vi "Odometry.vi"(0 "Enc0":dbl, 1 "Enc1":dbl, 2 "Enc2":dbl, 3 "Enc3":dbl, 4 "Az0":dbl, 5 "Az1":dbl, 6 "Az2":dbl, 7 "Az3":dbl, 8 "Heading":dbl, 9 "in SWERVE_DRIVE_ODOMETRY":T1={"POSE"={"TRANSLATION"={"X"=0.0, "Y"=0.0}, "ROTATION"={"VALUE"=0.0, "COS"=1.0, "SIN"=0.0}}, "GyroOffset"={"VALUE"=0.0, "COS"=1.0, "SIN"=0.0}, "PreviousAngle"={"VALUE"=0.0, "COS"=1.0, "SIN"=0.0}, "PrevModulePositions"=[], "NumModules"=0} {"PrevModulePositions"."Angle"."SIN" format="%13.4f"; "PrevModulePositions"."Angle"."COS" format="%13.4f"; "PrevModulePositions"."Angle"."VALUE" format="%13.4f"; "PreviousAngle"."SIN" format="%13.4f"; "PreviousAngle"."COS" format="%13.4f"; "PreviousAngle"."VALUE" format="%13.4f"; "GyroOffset"."SIN" format="%13.4f"; "GyroOffset"."COS" format="%13.4f"; "GyroOffset"."VALUE" format="%13.4f"; "POSE"."ROTATION"."SIN" format="%13.4f"; "POSE"."ROTATION"."COS" format="%13.4f"; "POSE"."ROTATION"."VALUE" format="%13.4f"; "POSE"."TRANSLATION"."Y" format="%14.3f"; "POSE"."TRANSLATION"."X" format="%14.3f"}) -> (20 "robot POSE":T2={"TRANSLATION"={"X"=0.0, "Y"=0.0}, "ROTATION"={"VALUE"=0.0, "COS"=1.0, "SIN"=0.0}} {"ROTATION"."SIN" format="%13.4f"; "ROTATION"."COS" format="%13.4f"; "ROTATION"."VALUE" format="%13.4f"; "TRANSLATION"."Y" format="%14.3f"; "TRANSLATION"."X" format="%14.3f"}, 21 "out SWERVE_DRIVE_ODOMETRY":T1={"POSE"={"TRANSLATION"={"X"=0.0, "Y"=0.0}, "ROTATION"={"VALUE"=0.0, "COS"=1.0, "SIN"=0.0}}, "GyroOffset"={"VALUE"=0.0, "COS"=1.0, "SIN"=0.0}, "PreviousAngle"={"VALUE"=0.0, "COS"=1.0, "SIN"=0.0}, "PrevModulePositions"=[], "NumModules"=0} {"PrevModulePositions"."Angle"."SIN" format="%13.4f"; "PrevModulePositions"."Angle"."COS" format="%13.4f"; "PrevModulePositions"."Angle"."VALUE" format="%13.4f"; "PreviousAngle"."SIN" format="%13.4f"; "PreviousAngle"."COS" format="%13.4f"; "PreviousAngle"."VALUE" format="%13.4f"; "GyroOffset"."SIN" format="%13.4f"; "GyroOffset"."COS" format="%13.4f"; "GyroOffset"."VALUE" format="%13.4f"; "POSE"."ROTATION"."SIN" format="%13.4f"; "POSE"."ROTATION"."COS" format="%13.4f"; "POSE"."ROTATION"."VALUE" format="%13.4f"; "POSE"."TRANSLATION"."Y" format="%14.3f"; "POSE"."TRANSLATION"."X" format="%14.3f"})   [LabVIEW 2020]
uses:
  <vilib>/Rock Robotics/WPI/ThirdParty/JAS_Junk/TrajLib/Trajectory_Library.lvlib
  <vilib>/Rock Robotics/WPI/ThirdParty/JAS_Junk/TrajLib/TypeDef/TRANSLATION2D.ctl
  <vilib>/Rock Robotics/WPI/ThirdParty/JAS_Junk/TrajLib/TypeDef/ROTATION2D.ctl
  <vilib>/Rock Robotics/WPI/ThirdParty/JAS_Junk/TrajLib/TypeDef/POSE2D.ctl
  <vilib>/Rock Robotics/WPI/ThirdParty/JAS_Junk/TrajLib/TypeDef/SWERVE_DRIVE_MODULE_POSITION.ctl
  <vilib>/Rock Robotics/WPI/ThirdParty/JAS_Junk/TrajLib/TypeDef/SWERVE_DRIVE_ODOMETRY.ctl
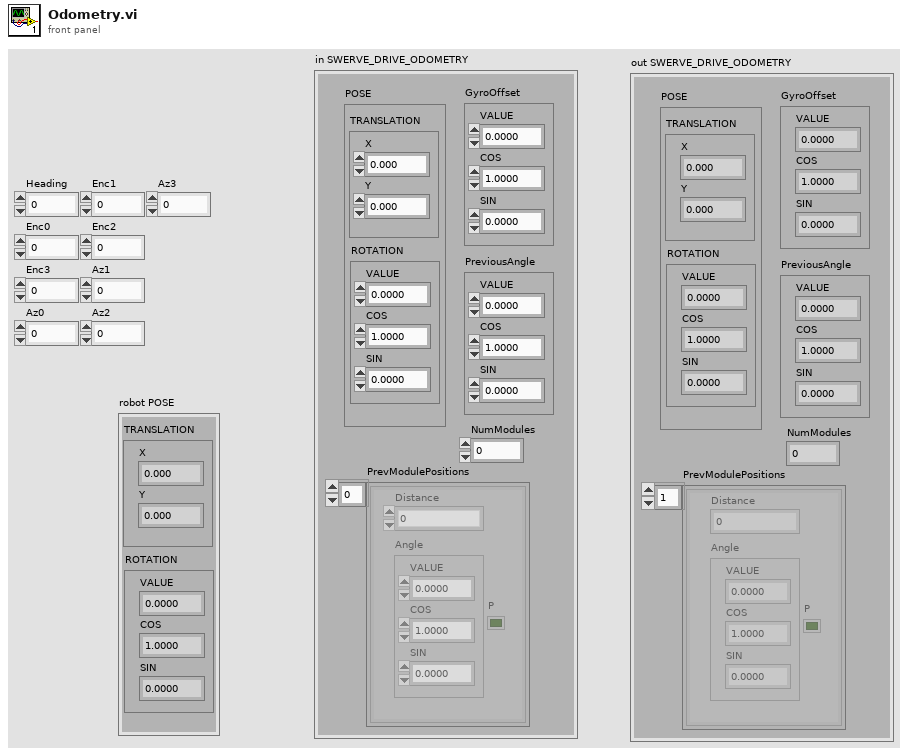
[diagram p1: front panel]
types:
  T1 = typedef "Trajectory_Library.lvlib/SWERVE_DRIVE_ODOMETRY.ctl" = cluster{"POSE":T2, "GyroOffset":T4, "PreviousAngle":T4, "PrevModulePositions":T5[], "NumModules":i32}
  T2 = typedef "Trajectory_Library.lvlib/POSE2D.ctl" = cluster{"TRANSLATION":T3, "ROTATION":T4}
  T3 = typedef "Trajectory_Library.lvlib/TRANSLATION2D.ctl" = cluster{"X":dbl, "Y":dbl}
  T4 = typedef "Trajectory_Library.lvlib/ROTATION2D.ctl" = cluster{"VALUE":dbl, "COS":dbl, "SIN":dbl}
  T5 = typedef "Trajectory_Library.lvlib/SWERVE_DRIVE_MODULE_POSITION.ctl" = cluster{"Distance":dbl, "Angle":T4, "P":bool}
  T6 = typedef "Trajectory_Library.lvlib/SWERVE_DRIVE_KINEMATICS.ctl" = cluster{"NumModules":i32, "InverseKinematics":T7, "ForwardKinematics":T7, "Modules":T3[], "PrevCoR":T3, "SavedModuleStates":T8[]}
  T7 = typedef "NI_Matrix.lvlib/RealMatrix.ctl" = dbl[][]
  T8 = typedef "Trajectory_Library.lvlib/SWERVE_DRIVE_MODULE_STATE.ctl" = cluster{"Speed":dbl, "Angle":T4}
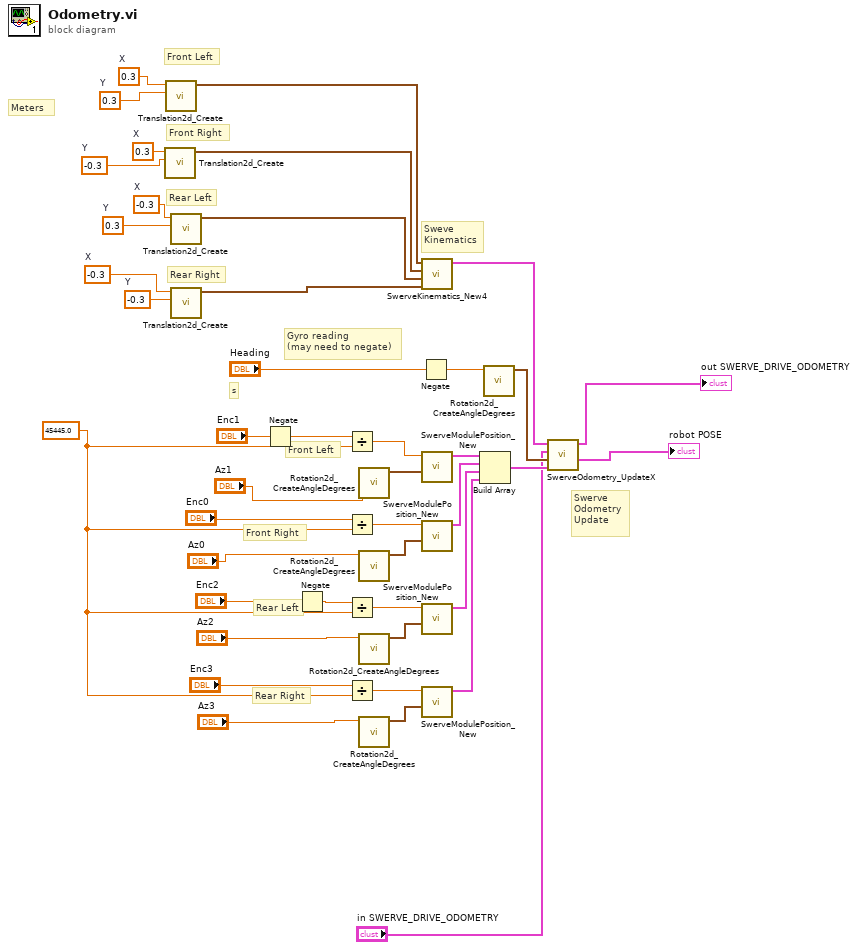
[diagram p0: block diagram]
diagram:
  w23 = 45445.0 ("y")
  w34 = -0.3  # X
  w35 = -0.3  # Y
  w32 = -0.3  # X
  w33 = 0.3  # Y
  w30 = 0.3  # X
  w31 = -0.3  # Y
  w28 = 0.3  # X
  w29 = 0.3  # Y
  # "s"
  # "Meters"
  # "Sweve\nKinematics"
  # "Rear Right"
  # "Rear Left"
  # "Front Right"
  # "Front Left"
  # "Swerve\nOdometry\nUpdate"
  # "Rear Right"
  # "Rear Left"
  # "Front Right"
  # "Front Left"
  # "Gyro reading\n(may need to negate)"
  n1 = call <vilib>:"Translation2d_Create.vi"("Y"=w31, "X"=w30) -> ("TRANSLATION"=w18:T3)  [unwired: 9 in]
  n2 = call <vilib>:"Translation2d_Create.vi"("Y"=w29, "X"=w28) -> ("TRANSLATION"=w19:T3)  [unwired: 9 in]
  n3 = call <vilib>:"Translation2d_Create.vi"("Y"=w33, "X"=w32) -> ("TRANSLATION"=w17:T3)  [unwired: 9 in]
  n4 = call <vilib>:"Translation2d_Create.vi"("Y"=w35, "X"=w34) -> ("TRANSLATION"=w16:T3)  [unwired: 9 in]
  n5 = Negate(x="Enc1") -> (-x=w2:dbl)
  n6 = Negate(x="Enc2") -> (-x=w1:dbl)
  n7 = Divide(x=w2, y=w23) -> (x/y=w27:dbl)
  n8 = Divide(x="Enc0", y=w23) -> (x/y=w26:dbl)
  n9 = Divide(x=w1, y=w23) -> (x/y=w25:dbl)
  n10 = Divide(x="Enc3", y=w23) -> (x/y=w24:dbl)
  n11 = call <vilib>:"Rotation2d_CreateAngleDegrees.vi"("Angle_Degrees"="Az1") -> ("ROTATION"=w40:T4)  [unwired: 10 in]
  n12 = call <vilib>:"Rotation2d_CreateAngleDegrees.vi"("Angle_Degrees"="Az0") -> ("ROTATION"=w41:T4)  [unwired: 10 in]
  n13 = call <vilib>:"Rotation2d_CreateAngleDegrees.vi"("Angle_Degrees"="Az2") -> ("ROTATION"=w42:T4)  [unwired: 10 in]
  n14 = call <vilib>:"Rotation2d_CreateAngleDegrees.vi"("Angle_Degrees"="Az3") -> ("ROTATION"=w43:T4)  [unwired: 10 in]
  n15 = Negate(x="Heading") -> (-x=w20:dbl)
  n16 = call <vilib>:"SwerveKinematics_New4.vi"("wheel 3"=w16, "wheel 2"=w17, "wheel 1"=w18, "wheel 0"=w19) -> ("SWERVE_DRIVE_KINEMATICS"=w10:T6)  [unwired: 7 in]
  n17 = call <vilib>:"SwerveModulePosition_New.vi"("ROTATION"=w40, "Distance"=w27) -> ("SWERVE_DRIVE_MODULE_POSITION"=w15:T5)  [unwired: 9 in]
  n18 = call <vilib>:"SwerveModulePosition_New.vi"("ROTATION"=w41, "Distance"=w26) -> ("SWERVE_DRIVE_MODULE_POSITION"=w14:T5)  [unwired: 9 in]
  n19 = call <vilib>:"SwerveModulePosition_New.vi"("ROTATION"=w42, "Distance"=w25) -> ("SWERVE_DRIVE_MODULE_POSITION"=w13:T5)  [unwired: 9 in]
  n20 = call <vilib>:"SwerveModulePosition_New.vi"("ROTATION"=w43, "Distance"=w24) -> ("SWERVE_DRIVE_MODULE_POSITION"=w12:T5)  [unwired: 9 in]
  n21 = Build Array(w15, w14, w13, w12) -> (w11:T5[])
  n22 = call <vilib>:"Rotation2d_CreateAngleDegrees.vi"("Angle_Degrees"=w20) -> ("ROTATION"=w9:T4)  [unwired: 10 in]
  n23 = call <vilib>:"SwerveOdometry_UpdateX.vi"("module Positions"=w11, "gyroAngle"=w9, "in SWERVE_DRIVE_ODOMETRY"="in SWERVE_DRIVE_ODOMETRY", "SWERVE_DRIVE_KINEMATICS"=w10) -> ("robot POSE"=→"robot POSE":T2, "out SWERVE_DRIVE_ODOMETRY"=→"out SWERVE_DRIVE_ODOMETRY":T1)  [unwired: 5 in, 1 out]
